vi "Create Waveforms.vi"(0 "RFFE RegReadExt Command in":refnum<class "RFFE RegReadExt Command.lvclass">, 5 "instrument handle in":refnum<k15>, 11 "error in (no error)":errorcluster) -> (4 "RFFE RegReadExt Command out":refnum<class "RFFE RegReadExt Command.lvclass">, 6 "instrument handle out":refnum<k15>, 15 "error out":errorcluster)   [LabVIEW 2018, in "MIPI RFFE API.lvlib" / "RFFE RegReadExt Command.lvclass"]
uses:
  RFFE RegReadExt Command.lvclass
  C:/Users/semoore/Projects/mipi-rffe-labview-oop/Command/RFFE Command.lvclass
  Command/RFFE Command.lvclass/RFFE Command.ctl
  Command/Get Pin.vi
  <instrlib>/niDigital/niDigital.llb/niDigital Create Capture Waveform (Serial).vi
  Extended Command/RFFE Extended Command.lvclass
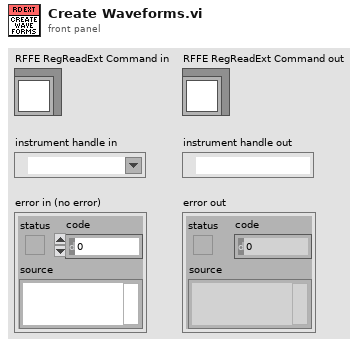
[diagram p1: front panel]
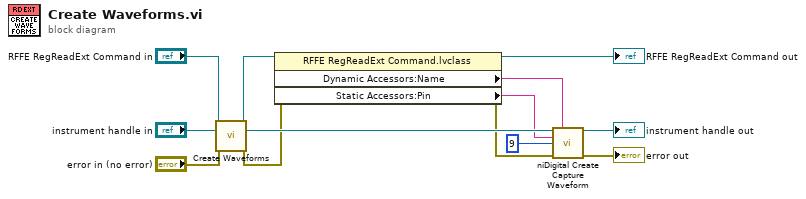
[diagram p0: block diagram]
diagram:
  n1 = call-parent "Create Waveforms.vi"("RFFE Command in"="RFFE RegReadExt Command in", "instrument handle in"="instrument handle in", "error in (no error)"="error in (no error)") -> ("RFFE Command out"=w9:refnum<class "RFFE RegReadExt Command.lvclass">, "instrument handle out"=w8:refnum<k15>, "error out"=w7:errorcluster)  [unwired: 10 in]
  n2 = property class="RFFE RegReadExt Command.lvclass"(reference=w9, error in=w7) -> (reference out=→"RFFE RegReadExt Command out":refnum<class "RFFE RegReadExt Command.lvclass">, error out=w1:errorcluster, "Dynamic Accessors:Name"=w3:string, "Static Accessors:Pin"=w2:string)
  n3 = call-poly <instrlib>:"niDigital Create Capture Waveform.vi"("instrument handle"=w8, "waveform name"=w3, "pin list"=w2, "sample width"=u32 9, "error in"=w1) -> ("instrument handle out"=→"instrument handle out":refnum<k15>, "error out"=→"error out":errorcluster)  [unwired: 9 in]
